vi "Test MQTT-3.2.2-4.vi"(8 "error in (no error)":errorcluster) -> (0 "error out":errorcluster)   [LabVIEW 2013]
uses:
  <vilib>/LabVIEW Open Source Project/MQTT Control Packets/Control Packets/CONNACK/Connect Return Code -- enum.ctl
  <vilib>/addons/_JKI Toolkits/Caraya/classes/Test/Test.lvclass
  <vilib>/LabVIEW Open Source Project/MQTT Control Packets/Control Packets/CONNACK/CONNACK.lvclass
  <vilib>/addons/_JKI Toolkits/Caraya/classes/Assert/Assert.lvclass
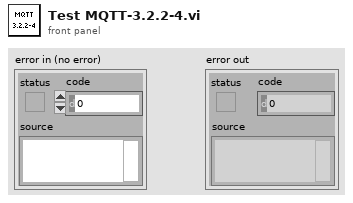
[diagram p1: front panel]
types:
  T1 = typedef "MQTT_Control_Packets.lvlib/CONNACK.lvclass/Connect Return Code -- enum.ctl" = enum16{"Connection accepted", "Unacceptable protocol version", "Identifier Rejected", "Server Unavailable", "Bad Username or Password", "Not Authorized"}
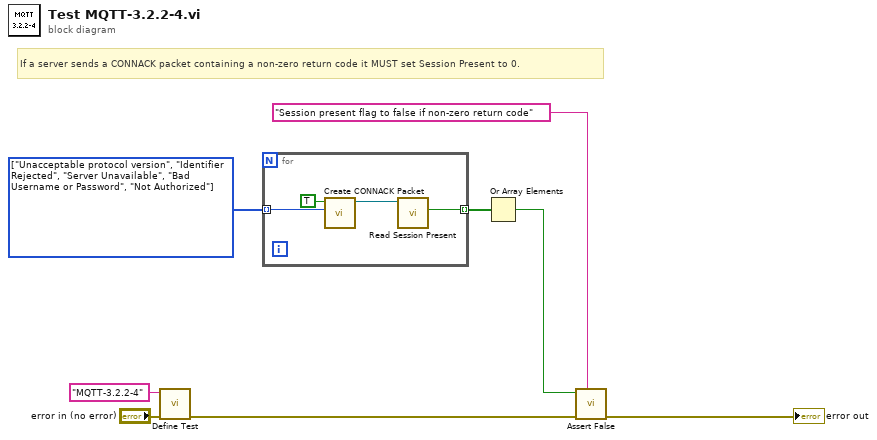
[diagram p0: block diagram]
diagram:
  w2 = T1[] [enum."Unacceptable protocol version", enum."Identifier Rejected", enum."Server Unavailable", enum."Bad Username or Password", enum."Not Authorized"] items=["Connection accepted", "Unacceptable protocol version", "Identifier Rejected", "Server Unavailable", "Bad Username or Password", "Not Authorized"]
  # "If a server sends a CONNACK packet containing a non-zero return code it MUST set Session Present to 0."
  n1 = call <vilib>:"Define Test.vi"("error in (no error)"="error in (no error)", "Label (VI Title)"="MQTT-3.2.2-4") -> ("error out"=w5:errorcluster)  [unwired: 9 in]
  n2 = for {
    tunnel: [w10] -> w3 mode=indexing
    tunnel: w2 -> [w9] mode=indexing
    n3 = call <vilib>:"Create CONNACK Packet.vi"("Return Code"=w9, "Session Present"=TRUE) -> ("CONNACK"=w11:refnum<class "CONNACK.lvclass">)  [unwired: 7 in, 2 out]
    n4 = call <vilib>:"Read Session Present.vi"("CONNACK in"=w11) -> ("Session Present"=w10:bool)  [unwired: 8 in, 2 out]
  }
  n5 = Or Array Elements(Boolean array=w3) -> (logical OR=w1:bool)
  n6 = call <vilib>:"Assert False.vi"("Label"="Session present flag to false if non-zero return code", "error in (no error)"=w5, "False?"=w1) -> ("error out"=→"error out":errorcluster)  [unwired: 8 in]
